vi "Test no to type.vi"(10 "number":dbl) -> (2 "String":string)   [LabVIEW 2011]
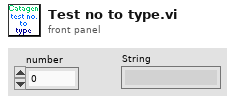
[diagram p1: front panel]
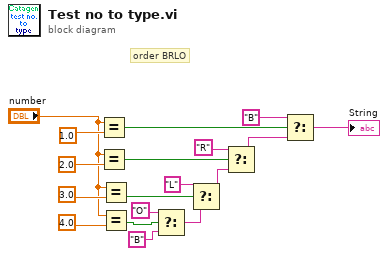
[diagram p0: block diagram]
diagram:
  # "order BRLO"
  n1 = Equal?(x="number", y=1.0 ("t")) -> (x = y?=w14:bool)
  n2 = Equal?(x="number", y=2.0 ("t")) -> (x = y?=w15:bool)
  n3 = Equal?(x="number", y=3.0 ("t")) -> (x = y?=w18:bool)
  n4 = Equal?(x="number", y=4.0 ("t")) -> (x = y?=w2:bool)
  n5 = Select(t="O", s=w2, f="B") -> (s? t:f=w4:string)
  n6 = Select(t="L", s=w18, f=w4) -> (s? t:f=w17:string)
  n7 = Select(t="R", s=w15, f=w17) -> (s? t:f=w16:string)
  n8 = Select(t="B", s=w14, f=w16) -> (s? t:f=→"String":string)
